vi "Get Data Channel Property - ALL.vi"(8 "error in":errorcluster, 11 "Item Ref in":T1 format="%.0x") -> (0 "error out":errorcluster, 2 "Item Informations array(parsed)":T2[](array[typedef]), 3 "Item Ref out":T1 format="%.0x")   [LabVIEW 2023, in "Vires VTD System Explorer.lvlib"]
uses:
  Vires VTD System Explorer.lvlib
  Item Informations.ctl
  <vilib>/NI VeriStand/Custom Device API/Custom Device Item Info.ctl
  <vilib>/NI VeriStand/Custom Device API/Custom Device Channel.ctl
  <vilib>/NI VeriStand/Custom Device API/Custom Device Channel Type.ctl
  Data Channel Custom Property.ctl
  <vilib>/NI VeriStand/Custom Device API/Custom Device Item Ref.ctl
  <vilib>/NI VeriStand/Custom Device API/Custom Device API.lvlib
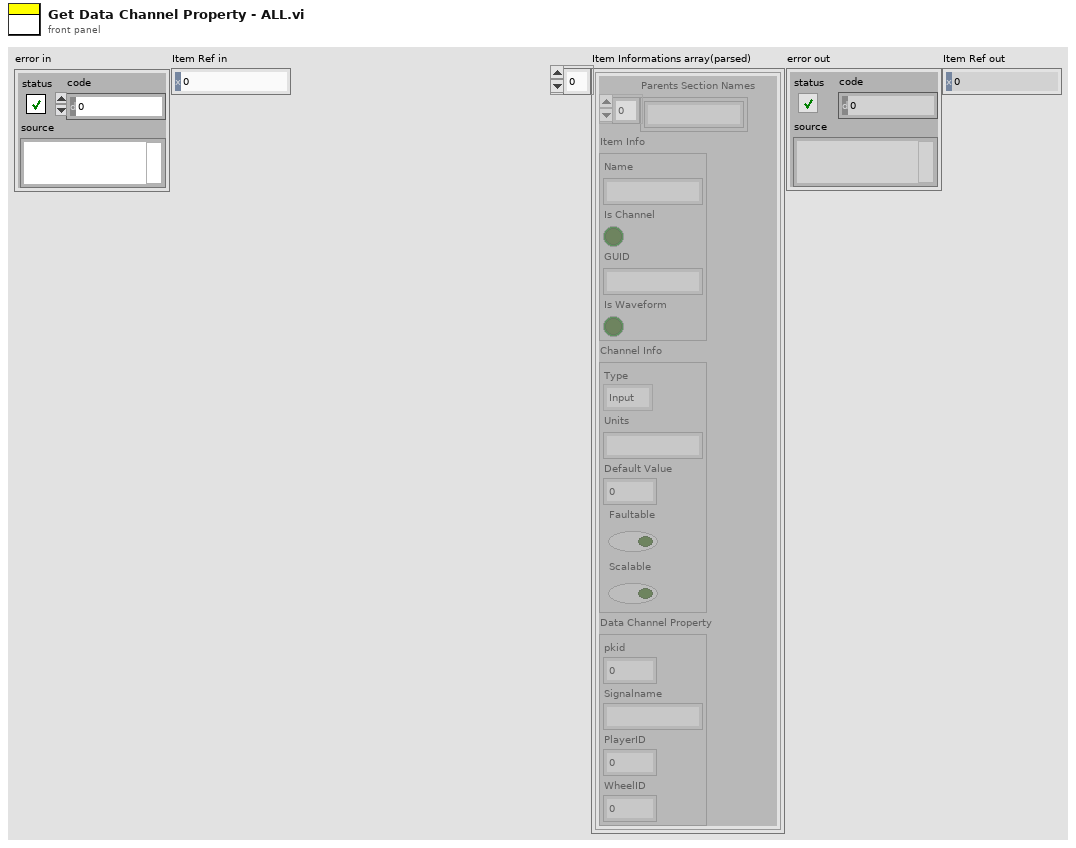
[diagram p1: front panel]
types:
  T1 = typedef "Custom Device API.lvlib/Custom Device Item Ref.ctl" = u64
  T2 = typedef "Vires VTD System Explorer.lvlib/Item Informations.ctl" = cluster{"Parents Section Names":string[], "Item Info":T3, "Channel Info":T4, "Data Channel Property":T6}
  T3 = typedef "Custom Device API.lvlib/Custom Device Item Info.ctl" = cluster{"Name":string, "Is Channel":bool, "GUID":string, "Is Waveform":bool}
  T4 = typedef "Custom Device API.lvlib/Custom Device Channel.ctl" = cluster{"Type":T5, "Units":string, "Default Value":dbl, "Faultable":bool, "Scalable":bool}
  T5 = typedef "Custom Device API.lvlib/Custom Device Channel Type.ctl" = enum16{"Input", "Output"}
  T6 = typedef "Vires VTD System Explorer.lvlib/Data Channel Custom Property.ctl" = cluster{"pkid":u32, "Signalname":string, "PlayerID":u8, "WheelID":i32}
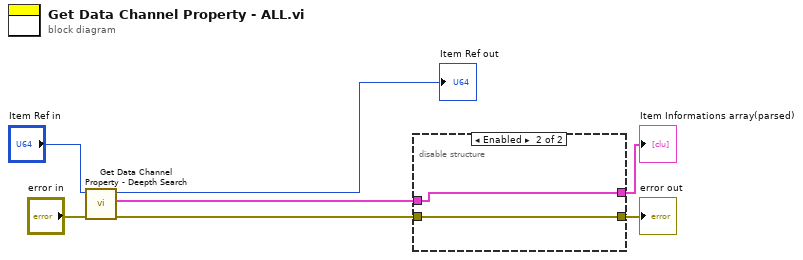
[diagram p0: block diagram]
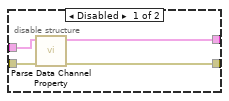
[diagram p2: hidden frame]
diagram:
  n1 = call "Get Data Channel Property - Deepth Search.vi"("error in"="error in", "Item Ref in"="Item Ref in") -> ("error out"=w2:errorcluster, "Item Informations array"=w7:T2[], "Item Ref out"=→"Item Ref out":T1)  [unwired: 7 in]
  n2 = disable-structure shown="Enabled" {
    disable-tunnel: w7 -> [w11 w13]
    disable-tunnel: [w10 w13] -> w6
    disable-tunnel: w2 -> [w9 w12]
    disable-tunnel: [w8 w12] -> w1
    frame Disabled {
      n3 = call "Parse Data Channel Property.vi"("error in (no error)"=w9, "Item Informations array"=w11) -> ("error out"=w8:errorcluster, "Item Informations array(parsed)"=w10:T2[])  [unwired: 8 in]
    }
    frame Enabled {
    }
  }
  "Item Informations array(parsed)" <- w6
  "error out" <- w1
